vi "fileIO_2.2.vi"() -> ()   [LabVIEW 2018]
panel:
  out "Usuarios":string[][](array[string])
  out "appended path":path
  in  "stop":bool
  out "Tab Control":T1(tab)
  in  "Ingresar":bool
  in  "Contraseña":string
  in  "usuario":string
  in  "Menu Agregar":bool
  in  "Menu Eliminar":bool
  in  "id_usuario":string
  in  "contrase_usuario":string
  in  "Agregar usuario":bool
  in  "Menú":bool
  in  "ID_usuario":string
  in  "contrase_usuario":string
  in  "Eliminar usuario":bool
  in  "Menú":bool
  in  "Cerrar cesión":bool
  out "usuario  ingresado":string
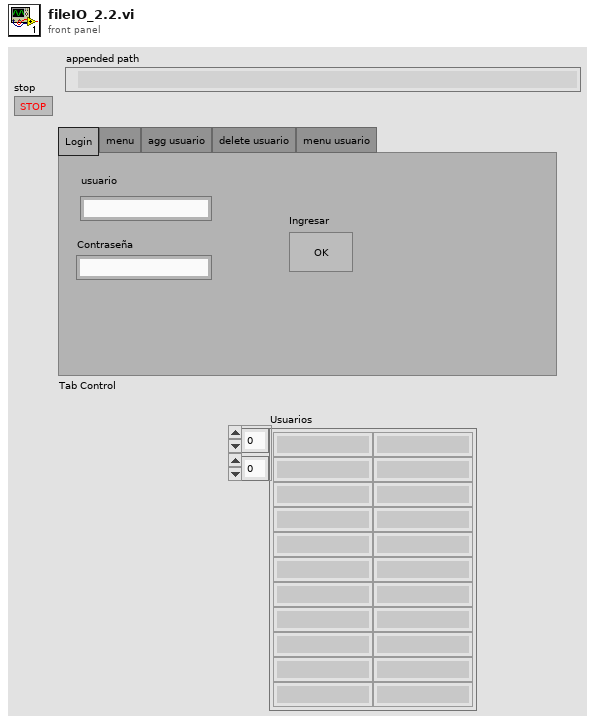
[diagram p1: front panel]
types:
  T1 = enum32{"Login", "menu", "agg usuario", "delete usuario", "menu usuario"}
  T2 = enum32{"Login", "menu", "agg usuario", "delete usuario"}
  T3 = enum16{"open", "replace", "create", "open or create", "replace or create", "replace or create with confirmation"}
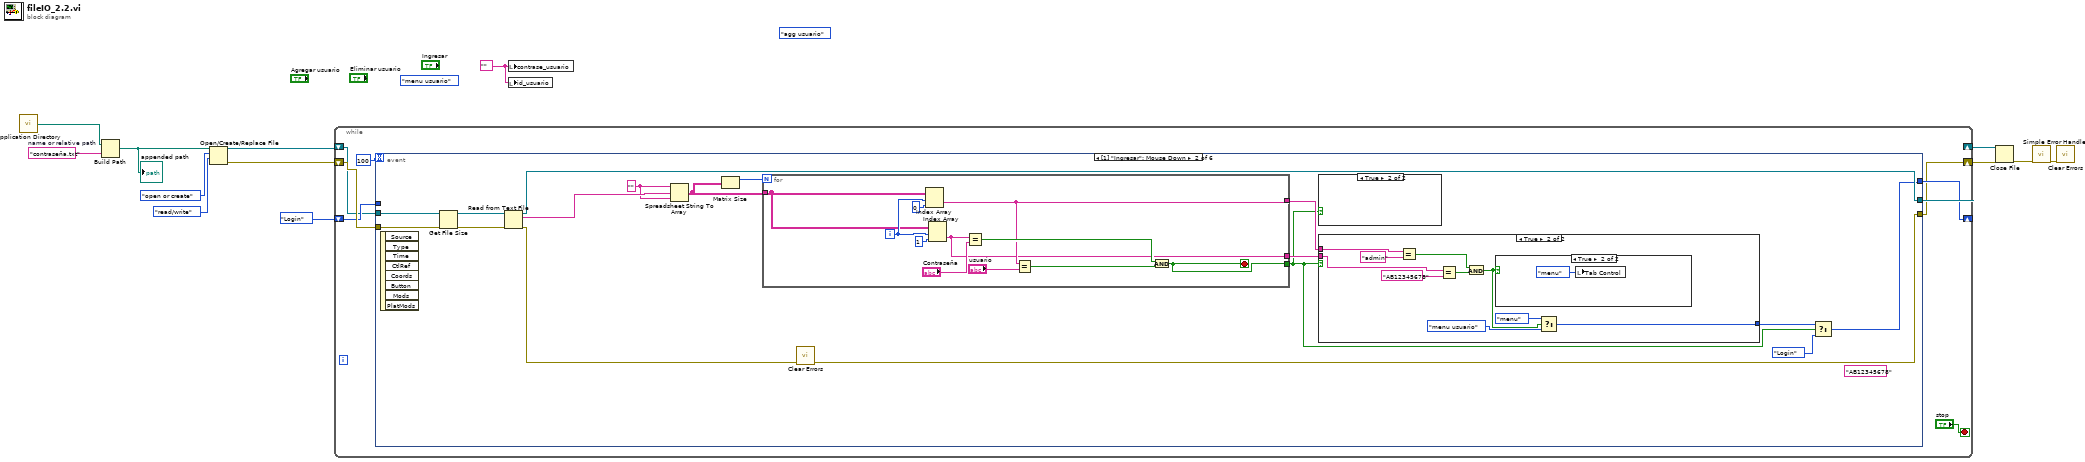
[diagram p0: block diagram]
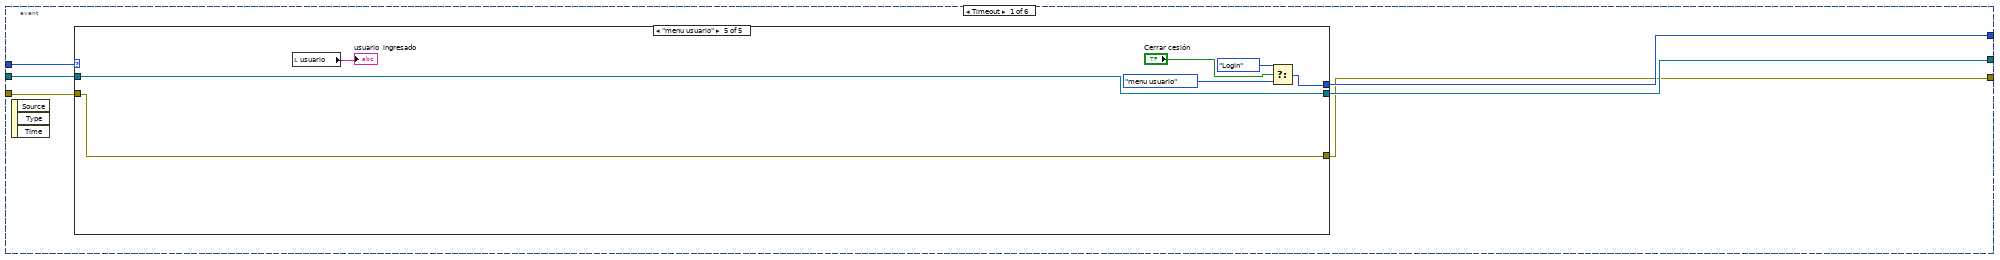
[diagram p2: hidden frame]
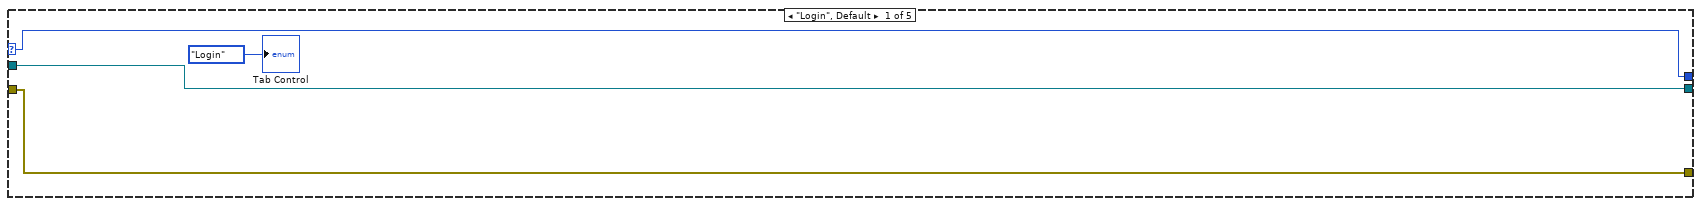
[diagram p3: hidden frame]
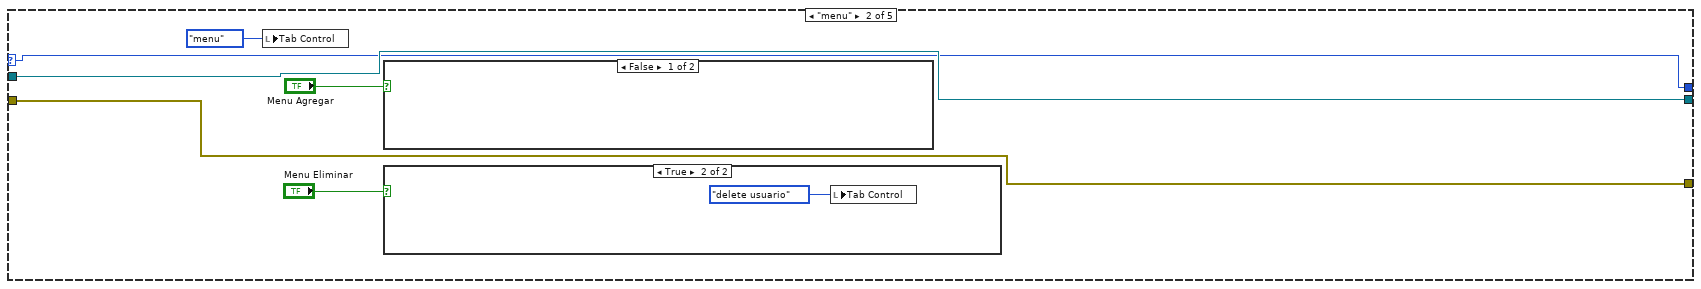
[diagram p4: hidden frame]
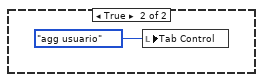
[diagram p6: hidden frame]
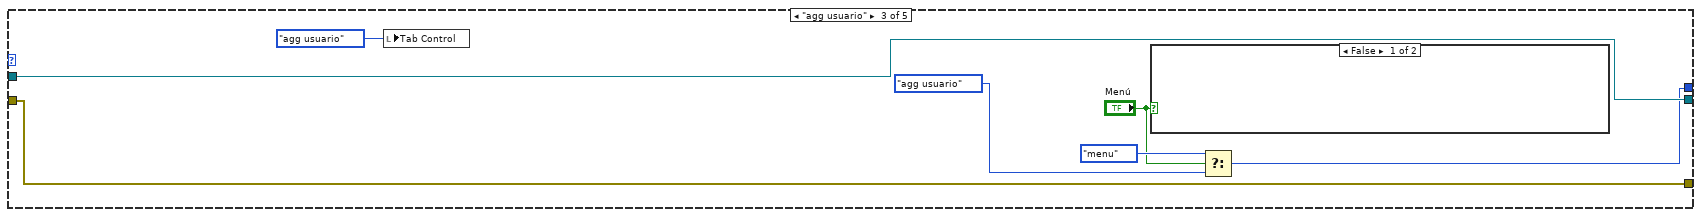
[diagram p7: hidden frame]
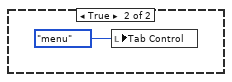
[diagram p8: hidden frame]
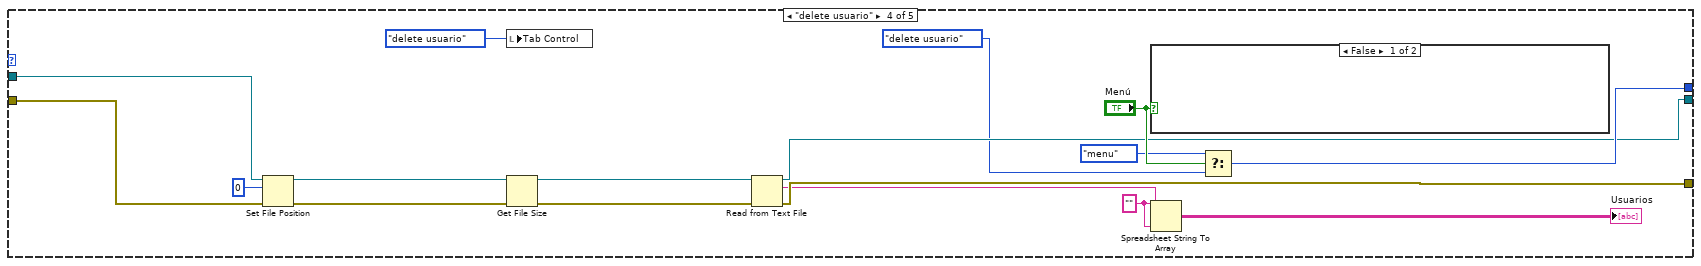
[diagram p9: hidden frame]
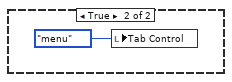
[diagram p10: hidden frame]
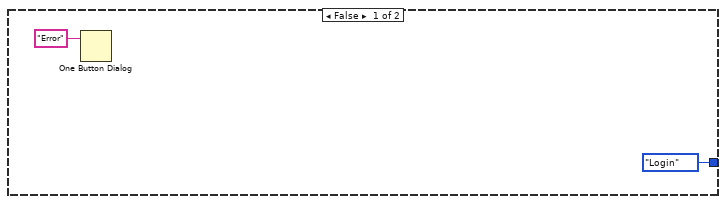
[diagram p11: hidden frame]
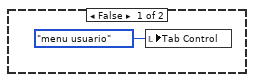
[diagram p12: hidden frame]
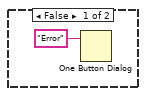
[diagram p13: hidden frame]
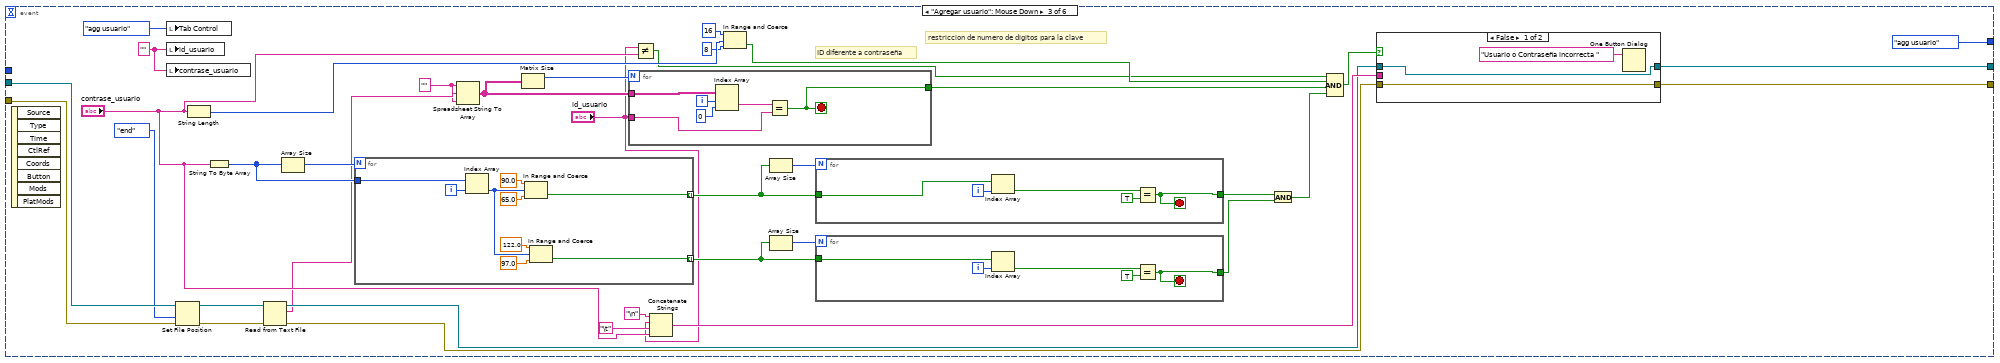
[diagram p14: hidden frame]
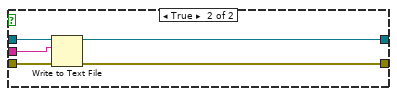
[diagram p15: hidden frame]
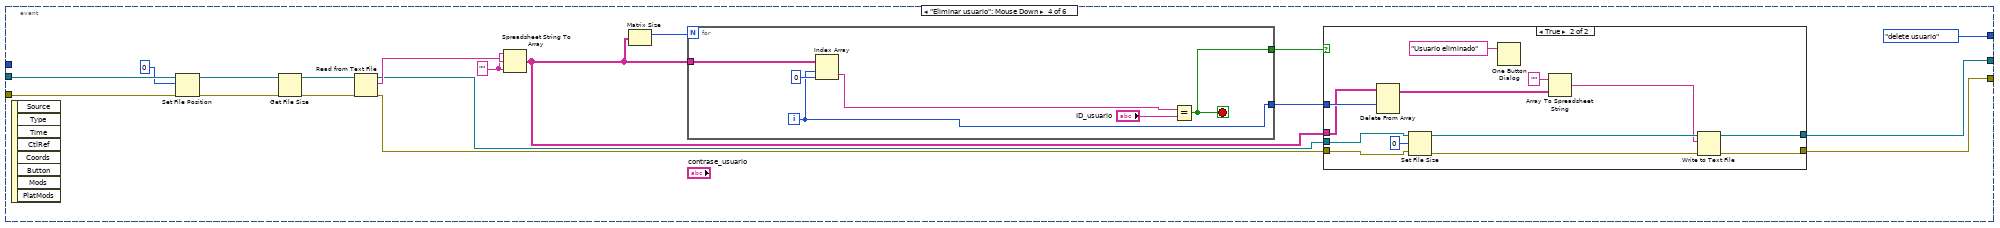
[diagram p16: hidden frame]
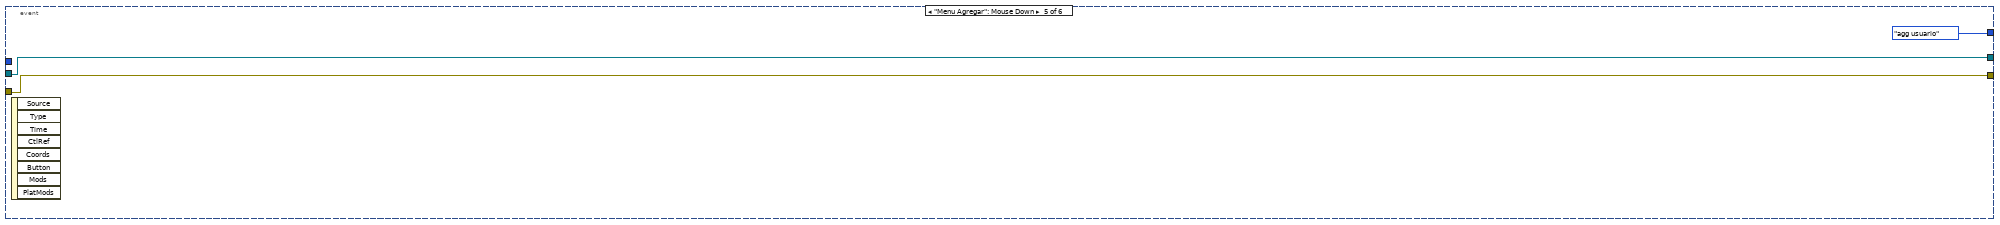
[diagram p18: hidden frame]
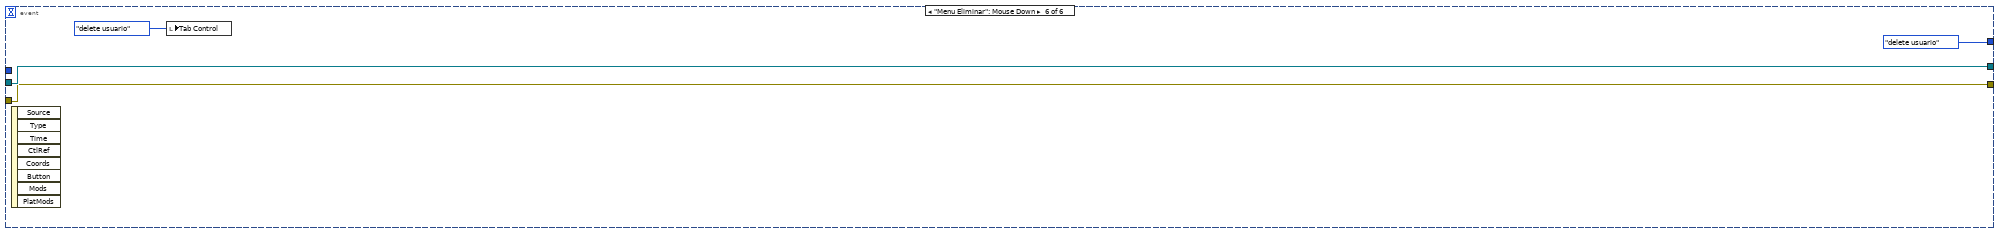
[diagram p19: hidden frame]
diagram:
  (unwired) T1."menu usuario" ("Tab Control")
  (unwired) T2."agg usuario" ("Tab Control")
  w5 = "" ("Contraseña")
  w12 = "contraseña.txt"  # name or relative path
  n1 = call <vilib>:"Application Directory.vi"() -> ("Application Directory"=w13:path)
  n2 = Build Path(base path=w13, name or relative path=w12) -> (appended path=w11:path)
  "appended path" <- w11
  n3 = Open/Create/Replace File(file path (use dialog)=w11, operation (0:open)=T3."open or create", access (0:read/write)=enum16{"read/write", "read-only", "write-only"}."read/write") -> (refnum out=w2:refnum<file>, error out=w4:errorcluster)  [unwired: 3 in, 1 out]
  n4 = while {
    shift-right: [w17] -> _
    shift-left: T1."Login" ("Tab Control") -> [w18]
    shift-right: [w15] -> w3
    shift-left: w4 -> [w21]
    shift-right: [w20] -> w6
    shift-left: w2 -> [w14]
    stop <- "stop" stop-if-true
    n5 = event shown="[1] \"Ingresar\": Mouse Down" {
      selector: _ -> [_ _ _ _ _ _]
      dyn-events: _ -> [_ _ _ _ _ _]
      timeout: 100 -> [_ _ _ _ _ _]
      tunnel: w14 -> [w26 w84 w152 w202 w225 w230]
      tunnel: w21 -> [w25 w85 w151 w201 w226 w229]
      tunnel: [w22 w88 w142 w187 w226 w229] -> w15
      tunnel: [w23 w87 w141 w188 w225 w230] -> w20
      tunnel: w18 -> [w27 _ _ _ _ _]
      tunnel: [w24 w86 T2."agg usuario" ("Tab Control") T2."delete usuario" ("Tab Control") T2."agg usuario" ("Tab Control") T2."delete usuario" ("Tab Control")] -> w17
      event Timeout {
        n6 = event-data() -> ()  [unwired: 1 in, 3 out]
        n7 = case shown="\"menu usuario\"" w27 {
          selector: w27 -> [w31 w35 _ _ _]
          tunnel: w26 -> [w30 w37 w46 w60 w72]
          tunnel: w25 -> [w29 w36 w45 w59 w71]
          tunnel: [w30 w37 w46 w62 w72] -> w23
          tunnel: [w29 w36 w45 w61 w71] -> w22
          tunnel: [w31 w35 w42 w64 w66] -> w24
          frame "Login", Default {
            "Tab Control" <- T1."Login" ("Tab Control")
          }
          frame "menu" {
            n8 = local write "Tab Control"(T1."menu" ("Tab Control")) -> ()
            n9 = case shown="False" "Menu Agregar" {
              frame False {
              }
              frame True {
                n10 = local write "Tab Control"(T2."agg usuario" ("Tab Control")) -> ()
              }
            }
            n11 = case shown="True" "Menu Eliminar" {
              frame False {
              }
              frame True {
                n12 = local write "Tab Control"(T1."delete usuario" ("Tab Control")) -> ()
              }
            }
          }
          frame "agg usuario" {
            n13 = local write "Tab Control"(T1."agg usuario" ("Tab Control")) -> ()
            n14 = case shown="False" "Menú" {
              frame False {
              }
              frame True {
                n15 = local write "Tab Control"(T2."menu" ("Tab Control")) -> ()
              }
            }
            n16 = Select(t=T2."menu" ("Tab Control"), s="Menú", f=T2."agg usuario" ("Tab Control")) -> (s? t:f=w42:T2)
          }
          frame "delete usuario" {
            w56 = "" ("format string")
            n17 = Set File Position(offset (in bytes) (0)=i64 0, refnum=w60, error in=w59) -> (refnum out=w55:refnum<file>, error out=w54:errorcluster)  [unwired: 1 in]
            n18 = local write "Tab Control"(T1."delete usuario" ("Tab Control")) -> ()
            n19 = Get File Size(file=w55, error in=w54) -> (refnum out=w53:refnum<file>, 0:w48:errorcluster)  [unwired: 1 out]
            n20 = Read from Text File(file (use dialog)=w53, error in=w48) -> (refnum out=w62:refnum<file>, text=w57:string, error out=w61:errorcluster)  [unwired: 2 in, 1 out]
            n21 = case shown="False" "Menú" {
              frame False {
              }
              frame True {
                n22 = local write "Tab Control"(T2."menu" ("Tab Control")) -> ()
              }
            }
            n23 = Spreadsheet String To Array(format string=w56, spreadsheet string=w57, array type (2D Dbl)=w56) -> (array=→"Usuarios":string[][])  [unwired: 1 in]
            n24 = Select(t=T1."menu" ("Tab Control"), s="Menú", f=T1."delete usuario" ("Tab Control")) -> (s? t:f=w64:T1)
          }
          frame "menu usuario" {
            n25 = local read "usuario"() -> (→"usuario  ingresado":string)
            n26 = Select(t=T1."Login" ("Tab Control"), s="Cerrar cesión", f=T1."menu usuario" ("Tab Control")) -> (s? t:f=w66:T1)
          }
        }
      }
      event "Ingresar": Mouse Down {
        w82 = "" ("format string")
        (unwired) "AB12345678" ("x")
        n27 = event-data() -> ()  [unwired: 1 in, 8 out]
        n28 = Get File Size(file=w84, error in=w85) -> (refnum out=w74:refnum<file>, 0:w73:errorcluster)  [unwired: 1 out]
        n29 = Read from Text File(file (use dialog)=w74, error in=w73) -> (refnum out=w87:refnum<file>, text=w83:string, error out=w89:errorcluster)  [unwired: 2 in, 1 out]
        n30 = Spreadsheet String To Array(format string=w82, spreadsheet string=w83, array type (2D Dbl)=w82) -> (array=w80:string[][])  [unwired: 1 in]
        n31 = Matrix Size(0:w80) -> (1:w81:i32)  [unwired: 1 out]
        n32 = for {
          N: w81 -> [_]
          tunnel: w80 -> [w111]
          tunnel: [w104] -> w77
          tunnel: [w106] -> w79
          tunnel: [w105] -> w78
          i -> [w113]
          stop <- w104 stop-if-true
          n33 = Index Array(array=w111, index (row)=w113, index (col)=0 ("index (row)")) -> (element=w106:string)
          n34 = Index Array(array=w111, index (row)=w113, index (col)=1) -> (element=w105:string)
          n35 = Equal?(x=w105, y="Contraseña") -> (x = y?=w109:bool)
          n36 = Equal?(x=w106, y="usuario") -> (x = y?=w108:bool)
          n37 = And(x=w109, y=w108) -> (x .and. y?=w104:bool)
        }
        n38 = call <vilib>:"Clear Errors.vi"("error in (no error)"=w89) -> ("error out"=w88:errorcluster)  [unwired: 5 in, 1 out]
        n39 = case shown="True" w77 {
          frame False {
            n40 = One Button Dialog(message="Error") -> ()  [unwired: 1 in, 1 out]
          }
          frame True {
          }
        }
        n41 = case shown="True" w77 {
          tunnel: w79 -> [_ w97]
          tunnel: w78 -> [_ w96]
          tunnel: [T1."Login" ("Tab Control") w92] -> w76
          frame False {
            n42 = One Button Dialog(message="Error") -> ()  [unwired: 1 in, 1 out]
          }
          frame True {
            n43 = Equal?(x=w97, y="admin") -> (x = y?=w98:bool)
            n44 = Equal?(x=w96, y="AB12345678") -> (x = y?=w101:bool)
            n45 = And(x=w98, y=w101) -> (x .and. y?=w95:bool)
            n46 = case shown="True" w95 {
              frame False {
                n47 = local write "Tab Control"(T1."menu usuario" ("Tab Control")) -> ()
              }
              frame True {
                n48 = local write "Tab Control"(T1."menu" ("Tab Control")) -> ()
              }
            }
            n49 = Select(t=T1."menu" ("Tab Control"), s=w95, f=T1."menu usuario" ("Tab Control")) -> (s? t:f=w92:T1)
          }
        }
        n50 = Select(t=w76, s=w77, f=T1."Login" ("Tab Control")) -> (s? t:f=w86:T1)
      }
      event "Agregar usuario": Mouse Down {
        w120 = "" ("format string")
        w148 = "" ("Contraseña")
        # "ID diferente a contraseña"
        # "restriccion de numero de digitos para la clave"
        n51 = event-data() -> ()  [unwired: 1 in, 8 out]
        n52 = local write "Tab Control"(T1."agg usuario" ("Tab Control")) -> ()
        n53 = local write "id_usuario"(w148) -> ()
        n54 = local write "contrase_usuario"(w148) -> ()
        n55 = Set File Position(refnum=w152, from (0:start)=enum16{"start", "end", "current"}."end", error in=w151) -> (refnum out=w125:refnum<file>, error out=w124:errorcluster)  [unwired: 1 in]
        n56 = String Length(string="contrase_usuario") -> (length=w147:i32)
        n57 = String To Byte Array(string="contrase_usuario") -> (unsigned byte array=w133:u8[])
        n58 = Read from Text File(file (use dialog)=w125, error in=w124) -> (refnum out=w123:refnum<file>, text=w121:string, error out=w122:errorcluster)  [unwired: 2 in, 1 out]
        n59 = Array Size(array=w133) -> (size(s)=w134:i32)
        n60 = for {
          N: w134 -> [_]
          tunnel: w133 -> [w177]
          tunnel: [w170] -> w131 mode=indexing
          tunnel: [w169] -> w127 mode=indexing
          i -> [w176]
          n61 = Index Array(array=w177, index=w176) -> (element=w171:u8)
          n62 = In Range and Coerce(upper limit=90.0, x=w171, lower limit=65.0) -> (In Range?=w170:bool)  [unwired: 1 out]
          n63 = In Range and Coerce(upper limit=122.0, x=w171, lower limit=97.0) -> (In Range?=w169:bool)  [unwired: 1 out]
        }
        n64 = Spreadsheet String To Array(format string=w120, spreadsheet string=w121, array type (2D Dbl)=w120) -> (array=w118:string[][])  [unwired: 1 in]
        n65 = Matrix Size(0:w118) -> (1:w119:i32)  [unwired: 1 out]
        n66 = for {
          N: w119 -> [_]
          tunnel: w118 -> [w158]
          tunnel: "id_usuario" -> [w154]
          tunnel: [w153] -> w116
          i -> [w156]
          stop <- w153 stop-if-true
          n67 = Index Array(array=w158, index (row)=w156, index (col)=0 ("disabled index (col)")) -> (element=w155:string)
          n68 = Equal?(x=w155, y=w154) -> (x = y?=w153:bool)
        }
        n69 = Not Equal?(x="id_usuario", y="contrase_usuario") -> (x != y?=w138:bool)
        n70 = Concatenate Strings("\n", "id_usuario", "\t", "contrase_usuario") -> (w143:string)
        n71 = In Range and Coerce(upper limit=16, x=w147, lower limit=8) -> (In Range?=w140:bool)  [unwired: 1 out]
        n72 = Array Size(array=w131) -> (size(s)=w130:i32)
        n73 = Array Size(array=w127) -> (size(s)=w126:i32)
        n74 = for {
          N: w130 -> [_]
          tunnel: w131 -> [w168]
          tunnel: [w164] -> w129
          i -> [w167]
          stop <- w164 stop-if-true
          n75 = Index Array(array=w168, index=w167) -> (element=w166:bool)
          n76 = Equal?(x=w166, y=TRUE) -> (x = y?=w164:bool)
        }
        n77 = for {
          N: w126 -> [_]
          tunnel: w127 -> [w163]
          tunnel: [w159] -> w128
          i -> [w162]
          stop <- w159 stop-if-true
          n78 = Index Array(array=w163, index=w162) -> (element=w161:bool)
          n79 = Equal?(x=w161, y=TRUE) -> (x = y?=w159:bool)
        }
        n80 = And(x=w129, y=w128) -> (x .and. y?=w132:bool)
        n81 = Compound Arithmetic op=AND(w138, w140, w116, w132) -> (w139:bool)
        n82 = case shown="False" w139 {
          tunnel: w123 -> [w179 w185]
          tunnel: w143 -> [_ w184]
          tunnel: [w178 w182] -> w142
          tunnel: [w179 w183] -> w141
          tunnel: w122 -> [w178 w181]
          frame False {
            n83 = One Button Dialog(message="Usuario o Contraseña incorrecta ") -> ()  [unwired: 1 in, 1 out]
          }
          frame True {
            n84 = Write to Text File(file (use dialog)=w185, text=w184, error in=w181) -> (refnum out=w183:refnum<file>, error out=w182:errorcluster)  [unwired: 1 in, 1 out]
          }
        }
      }
      event "Eliminar usuario": Mouse Down {
        w199 = "" ("format string")
        n85 = event-data() -> ()  [unwired: 1 in, 8 out]
        n86 = Set File Position(offset (in bytes) (0)=i64 0, refnum=w202, error in=w201) -> (refnum out=w193:refnum<file>, error out=w191:errorcluster)  [unwired: 1 in]
        n87 = Get File Size(file=w193, error in=w191) -> (refnum out=w192:refnum<file>, 0:w190:errorcluster)  [unwired: 1 out]
        n88 = Read from Text File(file (use dialog)=w192, error in=w190) -> (refnum out=w195:refnum<file>, text=w200:string, error out=w194:errorcluster)  [unwired: 2 in, 1 out]
        n89 = Spreadsheet String To Array(format string=w199, spreadsheet string=w200, array type (2D Dbl)=w199) -> (array=w186:string[][])  [unwired: 1 in]
        n90 = Matrix Size(0:w186) -> (1:w198:i32)  [unwired: 1 out]
        n91 = for {
          N: w198 -> [_]
          tunnel: [w220] -> w197
          tunnel: [w221] -> w196
          tunnel: w186 -> [w219]
          i -> [w221]
          stop <- w220 stop-if-true
          n92 = Index Array "Index Array"(array=w219, index (row)=w221, index (col)=0 ("disabled index (col)")) -> (element=w223:string)
          n93 = Equal?(x=w223, y="ID_usuario") -> (x = y?=w220:bool)
        }
        n94 = case shown="True" w197 {
          tunnel: w196 -> [_ w217]
          tunnel: w195 -> [w205 w214]
          tunnel: w194 -> [w204 w213]
          tunnel: [w205 w210] -> w188
          tunnel: [w204 w209] -> w187
          tunnel: w186 -> [_ w207]
          frame False {
          }
          frame True {
            n95 = Delete From Array "Delete From Array"(array=w207, index (row)=w217) -> (array with subset deleted=w206:string[][])  [unwired: 2 in, 1 out]
            n96 = Set File Size(4:w213, 6:i64 0 ("offset (in bytes) (0)"), 7:w214) -> (0:w211:errorcluster, 3:w212:refnum<file>)
            n97 = One Button Dialog(message="Usuario eliminado") -> ()  [unwired: 1 in, 1 out]
            n98 = Array To Spreadsheet String(array=w206, 3:"" ("format string")) -> (spreadsheet string=w208:string)  [unwired: 1 in]
            n99 = Write to Text File(file (use dialog)=w212, text=w208, error in=w211) -> (refnum out=w210:refnum<file>, error out=w209:errorcluster)  [unwired: 1 in, 1 out]
          }
        }
      }
      event "Menu Agregar": Mouse Down {
        n100 = event-data() -> ()  [unwired: 1 in, 8 out]
      }
      event "Menu Eliminar": Mouse Down {
        n101 = event-data() -> ()  [unwired: 1 in, 8 out]
        n102 = local write "Tab Control"(T1."delete usuario" ("Tab Control")) -> ()
      }
    }
  }
  n103 = local write "contrase_usuario"(w5) -> ()
  n104 = local write "id_usuario"(w5) -> ()
  n105 = Close File(refnum=w6, error in=w3) -> (error out=w8:errorcluster)  [unwired: 1 out]
  n106 = call <vilib>:"Simple Error Handler.vi"("error in (no error)"=w8) -> ("error out"=w7:errorcluster)  [unwired: 4 in, 4 out]
  n107 = call <vilib>:"Clear Errors.vi"("error in (no error)"=w7) -> ()  [unwired: 5 in, 2 out]
